vi "Done.vi"(8 "error in (no error)":errorcluster, 11 "Terminal Menus in":refnum<class "Terminal Menus.lvclass">) -> (0 "error out":errorcluster, 3 "Terminal Menus out":refnum<class "Terminal Menus.lvclass">)   [LabVIEW 2016, in "CLD Exam - ATM.lvlib" / "Terminal Menus.lvclass"]
uses:
  Terminal Menus.lvclass
  Mediator/Classes/Mediated Synchronous Actor/Mediated Synchronous Actor.lvclass
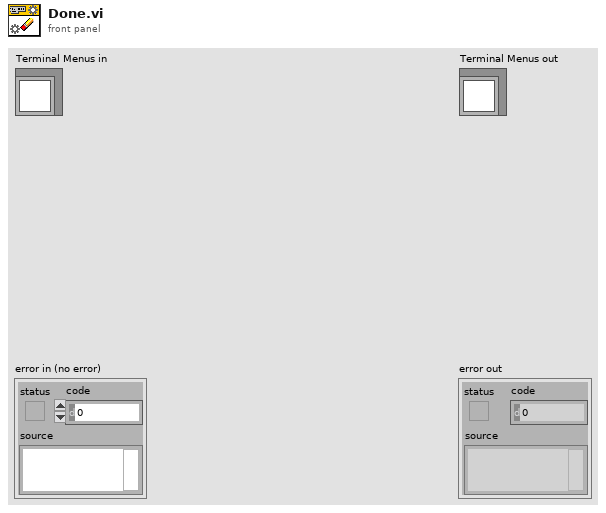
[diagram p1: front panel]
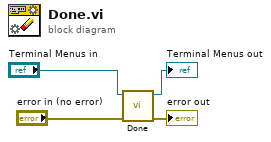
[diagram p0: block diagram]
diagram:
  n1 = call-parent "Done.vi"("error in (no error)"="error in (no error)", "Mediated Synchronous Actor in"="Terminal Menus in") -> ("error out"=→"error out":errorcluster, "Mediated Synchronous Actor out"=→"Terminal Menus out":refnum<class "Terminal Menus.lvclass">)  [unwired: 8 in]
